vi "Increment Error Counts.vi"(4 "specific errors":T4, 6 "receiving errors":i16, 7 "status error channel data references":T3 {"receiving" format="%.0x"; "specific errors"."gap" format="%.0x"; "specific errors"."parity" format="%.0x"; "specific errors"."long word" format="%.0x"; "specific errors"."bit timing" format="%.0x"; "specific errors"."timeout" format="%.0x"}, 8 "error in":errorcluster, 11 "error counts":T1) -> (0 "error out":errorcluster, 3 "error counts":T1)   [LabVIEW 2020, in "AIM ARINC 429 Engine.lvlib" / "Custom Device.lvlib"]
uses:
  Custom Device.lvlib
  <vilib>/NI VeriStand/Custom Device API/Data Reference.ctl
  <vilib>/NI VeriStand/Custom Device API/Global Data Refs.vi
  <vilib>/NI VeriStand/Custom Device API/Custom Device API.lvlib
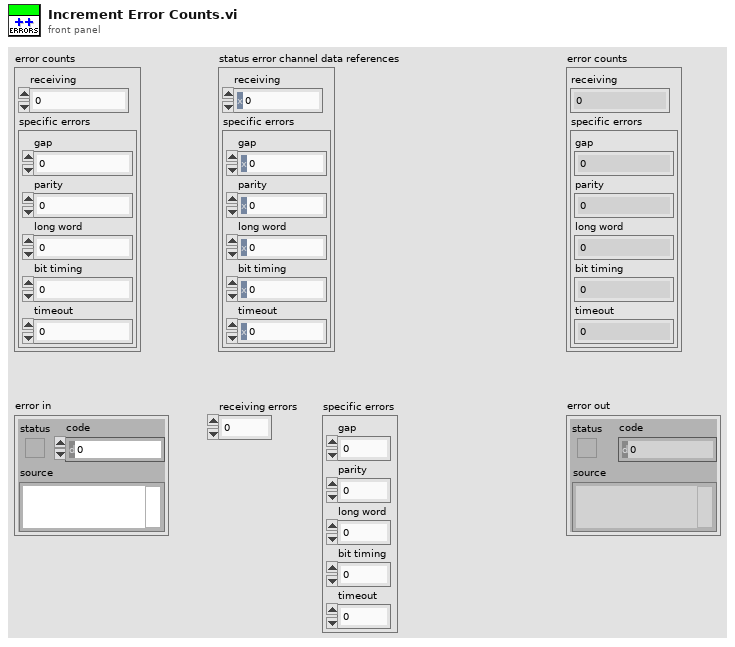
[diagram p1: front panel]
types:
  T1 = cluster{"receiving":dbl, "specific errors":cluster{"gap":dbl, "parity":dbl, "long word ":dbl, "bit timing":dbl, "timeout":dbl}}
  T2 = typedef "Custom Device API.lvlib/Data Reference.ctl" = i32
  T3 = cluster{"receiving":T2, "specific errors":cluster{"gap":T2, "parity":T2, "long word ":T2, "bit timing":T2, "timeout":T2}}
  T4 = cluster{"gap":i16, "parity":i16, "long word":i16, "bit timing":i16, "timeout":i16}
  T5 = cluster{"gap":dbl, "parity":dbl, "long word ":dbl, "bit timing":dbl, "timeout":dbl}
  T6 = cluster{"gap":dbl, "parity":dbl, "long word":dbl, "bit timing":dbl, "timeout":dbl}
  T7 = cluster{"gap":dbl, "parity":dbl, dbl, "bit timing":dbl, "timeout":dbl}
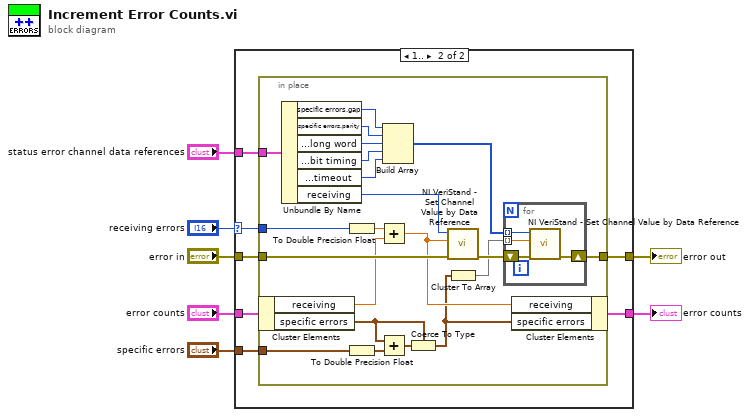
[diagram p0: block diagram]
diagram:
  n1 = case shown="1.." "receiving errors" {
    selector: "receiving errors" -> [_ w13]
    tunnel: [w9 w16] -> w7
    tunnel: "status error channel data references" -> [_ w15]
    tunnel: "specific errors" -> [_ w14]
    tunnel: "error in" -> [w9 w12]
    tunnel: "error counts" -> [w8 w11]
    tunnel: [w8 w10] -> w1
    frame Default {
    }
    frame 1.. {
      n2 = in-place {
        in-place-border: [w37] -> w16
        in-place-border: w15 -> [w36]
        in-place-border: w14 -> [w34]
        in-place-border: w13 -> [w33]
        in-place-border: w12 -> [w25]
        n3 = in-place-cluster #1(w11) -> ("receiving"=w22:dbl, "specific errors"=w20:T5)
        n4 = Unbundle By Name(w36) -> ("specific errors.gap"=w32:T2, "specific errors.parity"=w31:T2, "specific errors.long word"=w30:T2, "specific errors.bit timing"=w29:T2, "specific errors.timeout"=w28:T2, "receiving"=w26:T2)
        n5 = To Double Precision Float(number=w33) -> (double precision float=w24:dbl)
        n6 = To Double Precision Float(number=w34) -> (double precision float=w23:T6)
        n7 = Add(x=w24, y=w22) -> (x+y=w21:dbl)
        n8 = Add(x=w20, y=w23) -> (x+y=w19:T7)
        n9 = Build Array(w32, w31, w30, w29, w28) -> (w27:T2[])
        n10 = Coerce To Type(0:w19, 1:w20) -> (2:w18:T5)
        n11 = call <vilib>:"NI VeriStand - Set Channel Value by Data Reference.vi"("error in (no error)"=w25, "Value"=w21, "Data Reference in"=w26) -> ("error out"=w35:errorcluster)  [unwired: 8 in]
        n12 = Cluster To Array(cluster=w18) -> (array=w17:dbl[])
        n13 = for {
          shift-right: [w41] -> w37
          shift-left: w35 -> [w39]
          tunnel: w27 -> [w40] mode=indexing
          tunnel: w17 -> [w38] mode=indexing
          n14 = call <vilib>:"NI VeriStand - Set Channel Value by Data Reference.vi"("error in (no error)"=w39, "Value"=w38, "Data Reference in"=w40) -> ("error out"=w41:errorcluster)  [unwired: 8 in]
        }
        n15 = in-place-cluster #1("receiving"=w21, "specific errors"=w18) -> (w10:T1)
      }
    }
  }
  "error out" <- w7
  "error counts" <- w1
